vi "FRCts20_Backend_TeamList.vi"(8 "error in (no error)":errorcluster) -> (0 "error out":errorcluster, 3 "TeamList":T1)   [LabVIEW 2014, in "FRCts20_Backend_WebMethods.lvlib"]
doc: "The Get Team List Method will return a list of all teams registered with the FRCts 2.0 Service. The caller is provided <b>team number</b> and <b>location</b>."
uses:
  FRCts20_Backend_WebMethods.lvlib
  FRCts20_Backend_Engine.lvlib
  FRCts20_Backend_FGVOperation.ctl
  FRCts20_Backend_TeamList.ctl
  FRCts20_Backend_Controls.lvlib
panel:
  in  "TeamList Ref":T1
  # "The Get Team List Method will return a list of all\nteams registered with the FRCts 2.0 Service. The \ncaller is provided team number and location"
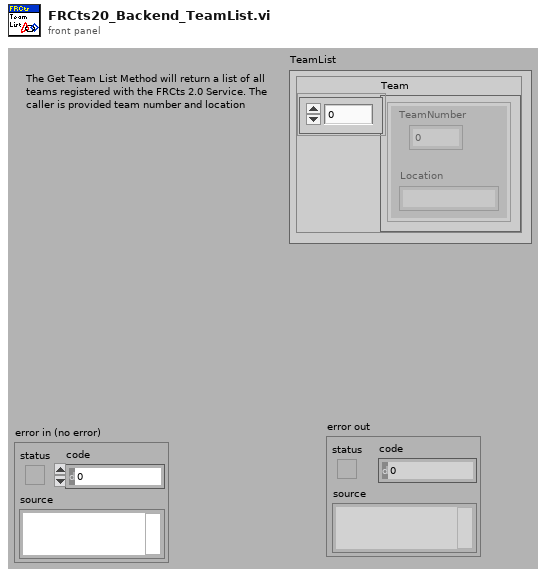
[diagram p1: front panel]
types:
  T1 = typedef "FRCts20_Backend_Controls.lvlib/FRCts20_Backend_TeamList.ctl" = cluster{"Team":cluster{"TeamNumber":u16, "Location":string}[]}
  T2 = typedef "FRCts20_Backend_Engine.lvlib/FRCts20_Backend_FGVOperation.ctl" = enum16{"Initialize", "EnqueueMessage", "EnqueueDataReturn", "FlushMessage", "FlushDataReturn"}
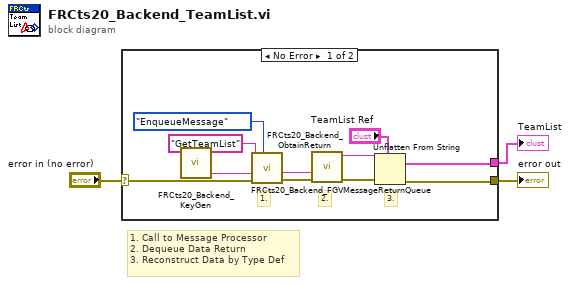
[diagram p0: block diagram]
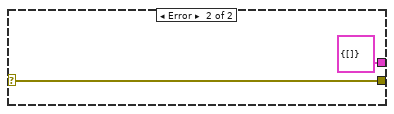
[diagram p2: hidden frame]
diagram:
  # "1. Call to Message Processor\n2. Dequeue Data Return\n3. Reconstruct Data by Type Def"
  n1 = case shown="No Error" "error in (no error)" {
    selector: "error in (no error)" -> [w14 w16]
    tunnel: [w6 w16] -> w2
    tunnel: [w7 T1 {"Team"=[]} ("TeamList 2")] -> w1
    frame No Error {
      # "3."
      # "2."
      # "1."
      n2 = call "FRCts20_Backend_KeyGen.vi"() -> ("Keygen"=w11:string)  [unwired: 27 in]
      n3 = call "FRCts20_Backend_FGVMessageReturnQueue.vi"("Operation"=FRCts20_Backend_FGVOperation."EnqueueMessage", "error in (no error)"=w14, "Key"=w11, "Message Name"="GetTeamList") -> ("error out"=w10:errorcluster, "Key (Duplicate)"=w5:string)  [unwired: 4 in]
      n4 = call "FRCts20_Backend_ObtainReturn.vi"("error in (no error)"=w10, "Key"=w5) -> ("error out"=w9:errorcluster, "Message Value"=w4:string)  [unwired: 8 in]
      n5 = Unflatten From String(type="TeamList Ref", binary string=w4, error in (no error)=w9) -> (value=w7:T1, error out=w6:errorcluster)  [unwired: 2 in, 1 out]
    }
    frame Error {
    }
  }
  "error out" <- w2
  "TeamList" <- w1
